vi "multimeter_measure.vi"(8 "error in (no error)":errorcluster, 9 "Switch 1000x":bool, 10 "Switch Multimeter":bool, 11 "VISA resource name":refnum<visa-resource-name>) -> (0 "error out":errorcluster, 1 "String":string, 2 "Reading":dbl format="%^.3e", 3 "VISA resource name out":refnum<visa-resource-name>)   [LabVIEW 2016]
uses:
  <instrlib>/Agilent 3446X Series/Public/Data/Read (Single Point).vi
  <instrlib>/Agilent 3446X Series/Agilent 3446X Series.lvlib
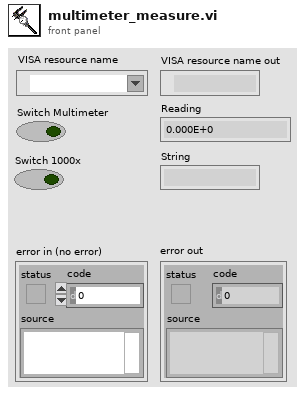
[diagram p1: front panel]
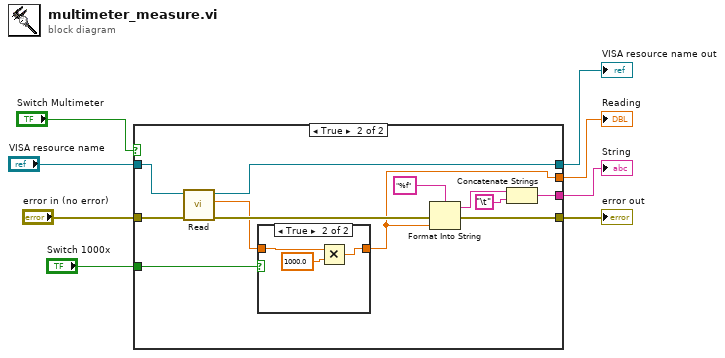
[diagram p0: block diagram]
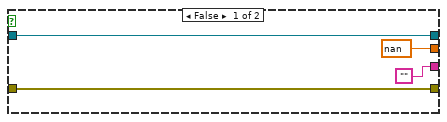
[diagram p2: hidden frame]
diagram:
  n1 = case shown="True" "Switch Multimeter" {
    tunnel: "VISA resource name" -> [w12 w24]
    tunnel: "error in (no error)" -> [w11 w23]
    tunnel: [w12 w22] -> w6
    tunnel: [nan ("Field Reading") w15] -> w5
    tunnel: [w11 w20] -> w2
    tunnel: ["" w16] -> w3
    tunnel: "Switch 1000x" -> [_ w13]
    frame False {
    }
    frame True {
      n2 = call-poly <instrlib>:"Read.vi"("error in (no error)"=w23, "VISA resource name"=w24) -> ("error out"=w21:errorcluster, "Measurement"=w14:dbl, "VISA resource name out"=w22:refnum<visa-resource-name>)  [unwired: 7 in]
      n3 = case shown="True" w13 {
        tunnel: [w25 w28] -> w15
        tunnel: w14 -> [w25 w27]
        frame False {
        }
        frame True {
          n4 = Multiply(x=w27, y=1000.0) -> (x*y=w28:dbl)
        }
      }
      n5 = Format Into String(format string="%f", error in=w21, w15) -> (resulting string=w18:string, error out=w20:errorcluster)  [unwired: 1 in]
      n6 = Concatenate Strings(w18, "\t") -> (w16:string)
    }
  }
  "VISA resource name out" <- w6
  "Reading" <- w5
  "error out" <- w2
  "String" <- w3
